vi "FNV-32 bit.vi"(2 "Key":string) -> (16 "32 bit FNV-1 hash":u32 format="%x")   [LabVIEW 2012]
doc: "32 bit Fowler-Noll-Vo hash function\n\nhttp://en.wikipedia.org/wiki/Fowler%E2%80%93Noll%E2%80%93Vo_hash_function\n\nImplementation by Mads A. Toppe."
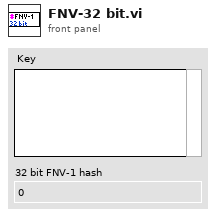
[diagram p1: front panel]
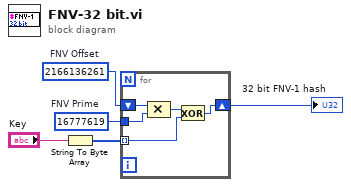
[diagram p0: block diagram]
diagram:
  w4 = u32 16777619  # FNV Prime
  w5 = u32 2166136261  # FNV Offset
  n1 = String To Byte Array(string="Key") -> (unsigned byte array=w1:u8[])
  n2 = for {
    shift-right: [w7] -> w3
    shift-left: w5 -> [w10]
    tunnel: w4 -> [w9]
    tunnel: w1 -> [w6] mode=indexing
    n3 = Compound Arithmetic op=MULTIPLY(w10, w9) -> (w8:u32)
    n4 = Exclusive Or(1:w6, 2:w8) -> (0:w7:u32)
  }
  "32 bit FNV-1 hash" <- w3
